vi "myFFT_abc2alphabeta.vi"(2 "C wave":dbl[](array[numeric]), 3 "B wave":dbl[](array[numeric]), 4 "A wave":dbl[](array[numeric])) -> (0 "beta wave":dbl[](array[numeric]), 1 "alpha wave":dbl[](array[numeric]))   [LabVIEW 2024]
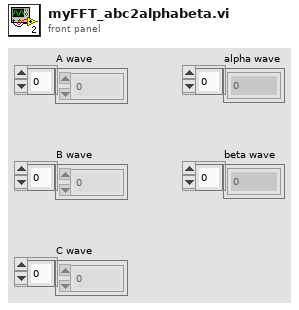
[diagram p1: front panel]
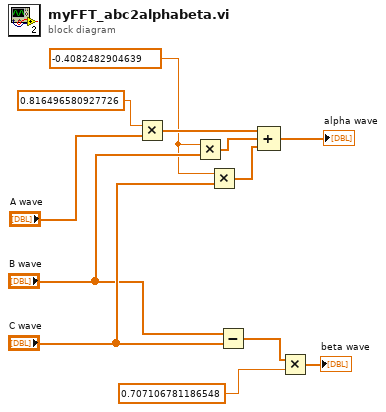
[diagram p0: block diagram]
diagram:
  w3 = -0.4082482904639
  n1 = Multiply(x=0.816496580927726, y="A wave") -> (x*y=w6:dbl[])
  n2 = Multiply(x=w3, y="B wave") -> (x*y=w5:dbl[])
  n3 = Multiply(x=w3, y="C wave") -> (x*y=w4:dbl[])
  n4 = Subtract(x="B wave", y="C wave") -> (x-y=w11:dbl[])
  n5 = Compound Arithmetic op=ADD(w6, w5, w4) -> (→"alpha wave":dbl[])
  n6 = Multiply(x=w11, y=0.707106781186548) -> (x*y=→"beta wave":dbl[])
